vi "Launch Controller.vi"(8 "error in (no error)":errorcluster, 10 "LVProjPath":path=path "", 11 "StatusQueue":refnum<queue>) -> (0 "error out":errorcluster)   [LabVIEW 2013, in "SET Project Editor.lvlib"]
doc: "Launch Controller.vi\n\nRunning this VI will start the SET Project Editor. Optional input parameters are:\n- StatusQueue: String queue from splash screen. Controller can use this queue to control the splash screen.\n- LVProjPath: Path to a \".lvproj\" file. Default value is <not a path>."
uses:
  <vilib>/ActorFramework/Message Queue/Message Queue.lvclass/Message Queue.ctl
  SET Project Editor.lvlib
  <vilib>/ActorFramework/Message Queue/Message Queue.lvclass
  <vilib>/ActorFramework/Actor/Actor.lvclass
  Controller/Controller.lvclass
  SET Project Data/SET Project Data.lvlib
panel:
  # "Launch Controller.vi\n\nRunning this VI will start the SET Project Editor. Optional input parameters are:\n- StatusQueue: String queue from splash screen. Controller can use this queue to control the splash screen.\n- LVProjPath: Path to a \".lvproj\" file. Default value is <not a path>."
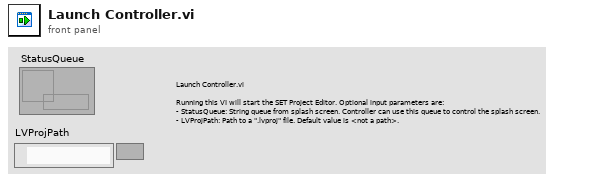
[diagram p1: front panel]
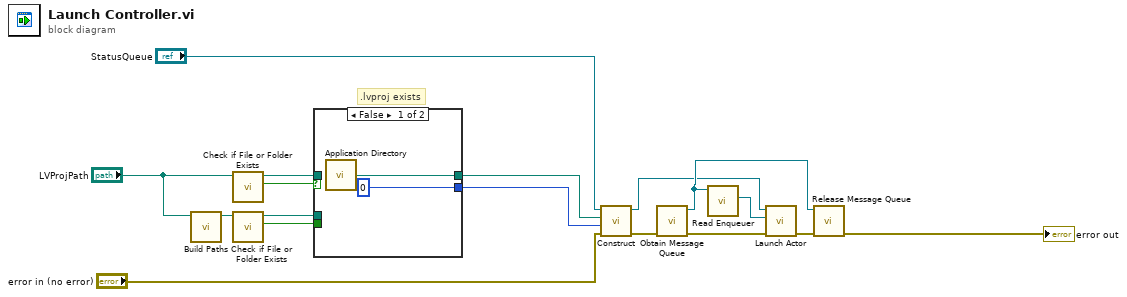
[diagram p0: block diagram]
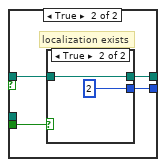
[diagram p2: hidden frame]
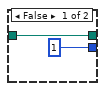
[diagram p3: hidden frame]
diagram:
  # ".lvproj exists"
  n1 = call "Build Paths.vi"("lvproj Path"="LVProjPath") -> ("SET ProjFile Path"=w10:path)  [unwired: 10 in]
  n2 = call <vilib>:"Check if File or Folder Exists.vi"("path"="LVProjPath") -> ("file or folder exists?"=w4:bool, "dup path"=w11:path)  [unwired: 8 in, 1 out]
  n3 = call <vilib>:"Check if File or Folder Exists.vi"("path"=w10) -> ("file or folder exists?"=w7:bool, "dup path"=w8:path)  [unwired: 8 in, 1 out]
  n4 = case shown="False" w4 {
    tunnel: w11 -> [_ w22]
    tunnel: w8 -> [_ _]
    tunnel: w7 -> [_ w23]
    tunnel: [w19 w21] -> w6
    tunnel: [0 ("Launch Type (0)") w20] -> w5
    frame False {
      n5 = call <vilib>:"Application Directory.vi"() -> ("Application Directory"=w19:path)
    }
    frame True {
      # "localization exists"
      n6 = case shown="True" w23 {
        tunnel: w22 -> [w24 w27]
        tunnel: [w24 w27] -> w21
        tunnel: [1 ("t") 2 ("t")] -> w20
        frame False {
        }
        frame True {
        }
      }
    }
  }
  n7 = call "Construct.vi"("error in (no error)"="error in (no error)", "Launch Type (0)"=w5, "Default Path"=w6, "StatusQueue"="StatusQueue") -> ("error out"=w14:errorcluster, "Controller out"=w13:refnum<class "Controller.lvclass">)  [unwired: 6 in]
  n8 = call <vilib>:"Obtain Message Queue.vi"("error in (no error)"=w14) -> ("error out"=w17:errorcluster, "Message Queue"=w15:refnum<class "Message Queue.lvclass">)  [unwired: 9 in]
  n9 = call <vilib>:"Read Enqueuer.vi"("Message Queue"=w15) -> ("Message Enqueuer"=w16:refnum<class "Message Enqueuer.lvclass">)  [unwired: 10 in]
  n10 = call <vilib>:"Launch Actor.vi"("error in (no error)"=w17, "Actor-to-Caller Enqueuer"=w16, "Actor"=w13) -> ("error out"=w12:errorcluster)  [unwired: 7 in, 1 out]
  n11 = call <vilib>:"Release Message Queue.vi"("error in (no error)"=w12, "Message Queue"=w15) -> ("error out"=→"error out":errorcluster)  [unwired: 8 in, 1 out]
